vi "GA_Increment_NumberofJobsOn Machine_ByOne.vi"(10 "Machine Number":i32, 11 "Number of Jobs Scheduled On Machines in":i32[](array[numeric])) -> (3 "Number of Jobs Scheduled On Machines out":i32[](array[numeric]))   [LabVIEW 2013, in "GA.lvclass"]
uses:
  GA.lvclass
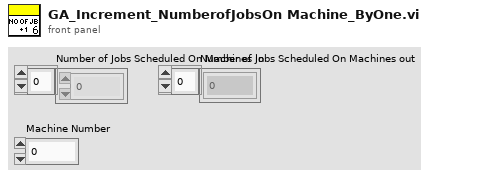
[diagram p1: front panel]
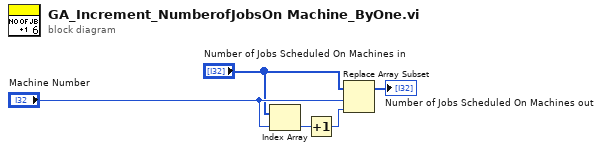
[diagram p0: block diagram]
diagram:
  n1 = Index Array(array="Number of Jobs Scheduled On Machines in", index="Machine Number") -> (element=w2:i32)
  n2 = Increment(x=w2) -> (x+1=w1:i32)
  n3 = Replace Array Subset(array="Number of Jobs Scheduled On Machines in", new element=w1, index="Machine Number") -> (→"Number of Jobs Scheduled On Machines out":i32[])
